vi "VCS Get Key Handle.vi"(8 "error in (no error)":errorcluster, 10 "device in":T1={"deviceName"="EPOS2", "protocolStackName"="", "interfaceName"="", "portName"=""}, 11 "axis in":cluster{"keyHandle":u32, "nodeId":u16}={"keyHandle"=0, "nodeId"=1}) -> (0 "error out":errorcluster, 2 "keyHandle":u32, 3 "axis out":cluster{"keyHandle":u32, "nodeId":u16}={"keyHandle"=0, "nodeId"=1})   [LabVIEW 2010]
doc: "<B>VCS Get Key Handle</B> returns the key handle."
uses:
  Resources/EposCmd.dll
  Resources/EposCmd64.dll
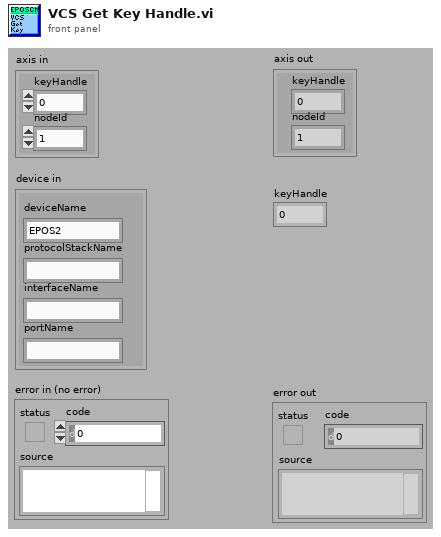
[diagram p1: front panel]
types:
  T1 = cluster{"deviceName":string, "protocolStackName":string, "interfaceName":string, "portName":string}
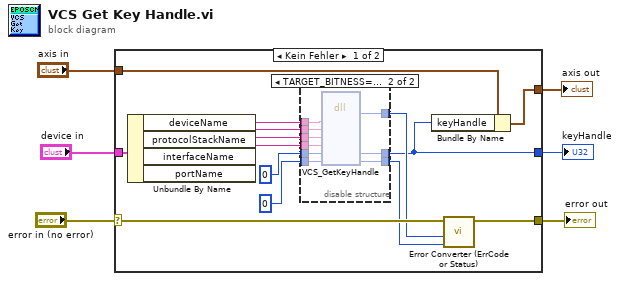
[diagram p0: block diagram]
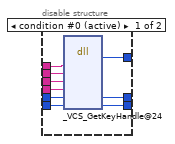
[diagram p2: hidden frame]
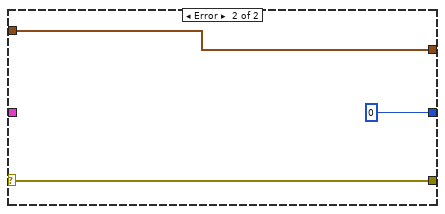
[diagram p3: hidden frame]
diagram:
  n1 = case shown="Kein Fehler" "error in (no error)" {
    selector: "error in (no error)" -> [w20 w41]
    tunnel: [w19 w41] -> w5
    tunnel: "device in" -> [w16 _]
    tunnel: "axis in" -> [w11 w40]
    tunnel: [w8 w40] -> w2
    tunnel: [w7 u32 0 ("pKeyHandle")] -> w1
    frame No Error {
      n2 = Unbundle By Name(w16) -> ("deviceName"=w15:string, "protocolStackName"=w14:string, "interfaceName"=w13:string, "portName"=w12:string)
      n3 = disable-structure shown="TARGET_BITNESS==64" {
        disable-tunnel: [w29 w38] -> w18
        disable-tunnel: [w28 w37] -> w17
        disable-tunnel: w15 -> [w27 w36]
        disable-tunnel: w14 -> [w26 w35]
        disable-tunnel: w13 -> [w25 w34]
        disable-tunnel: w12 -> [w24 w33]
        disable-tunnel: u32 0 ("pKeyHandle") -> [w23 w32]
        disable-tunnel: u32 0 ("pErrorCode") -> [w22 w31]
        disable-tunnel: [w21 w30] -> w7
        frame condition #0 (active) {
          n4 = dll-call lib="C:/Sources/LabView/maxon EPOS/Resources/EposCmd.*" fn="_VCS_GetKeyHandle@24"("DeviceName"=w27, "ProtocolStackName"=w26, "InterfaceName"=w25, "PortName"=w24, "pKeyHandle"=w23, "pErrorCode"=w22) -> (w29:i32, "pKeyHandle"=w21:u32, "pErrorCode"=w28:u32)  [unwired: 7 in, 2 out]
        }
        frame condition #1 {
          n5 = dll-call lib="C:/setup/Resources/EposCmd64.*" fn="VCS_GetKeyHandle" ("EposCmd.dll:_VCS_GetKeyHandle@24")("DeviceName"=w36, "ProtocolStackName"=w35, "InterfaceName"=w34, "PortName"=w33, "pKeyHandle"=w32, "pErrorCode"=w31) -> ("Rückgabetyp"=w38:i32, "pKeyHandle"=w30:u32, "pErrorCode"=w37:u32)  [unwired: 7 in, 2 out]
        }
      }
      n6 = Bundle By Name(cluster=w11, "keyHandle"=w7) -> (w8:cluster{"keyHandle":u32, "nodeId":u16})
      n7 = call "Error Converter (ErrCode or Status).vi"("error code"=w17, "return type"=w18, "error in (no error)"=w20) -> ("error out"=w19:errorcluster)  [unwired: 7 in]
    }
    frame Error {
    }
  }
  "error out" <- w5
  "axis out" <- w2
  "keyHandle" <- w1
